vi "result text16be.vi"(7 "para3":u32, 8 "error in (no error)":errorcluster, 9 "para2":i32, 10 "para1":u32, 11 "para0":dbl) -> (0 "error out":errorcluster, 3 "para0 out":dbl, 5 "para3 out":u32)   [LabVIEW 2020, in "sqlite3.lvlib"]
uses:
  sqlite3.lvlib
  errstr.vi
  bin/sqlite3_64.dll
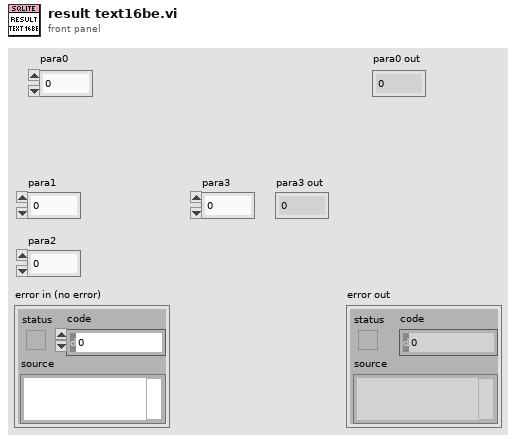
[diagram p1: front panel]
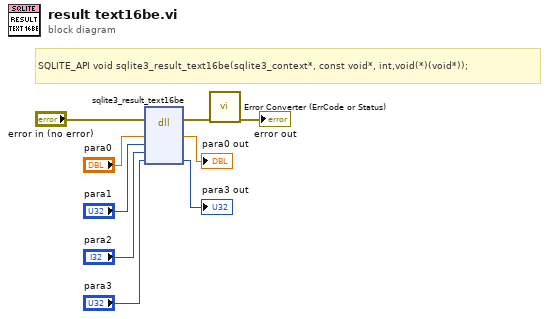
[diagram p0: block diagram]
diagram:
  # "SQLITE_API void sqlite3_result_text16be(sqlite3_context*, const void*, int,void(*)(void*));"
  n1 = dll-call lib="D:/Project/Labview-Projects/database-configuration/externals/sqlite3/Source/bin/sqlite3_*.*" fn="sqlite3_result_text16be"(error in="error in (no error)", "para0"="para0", "para1"="para1", "para2"="para2", "para3"="para3") -> (error out=w2:errorcluster, "para0"=→"para0 out":dbl, "para3"=→"para3 out":u32)  [unwired: 5 in, 1 out]
  n2 = call "Error Converter (ErrCode or Status).vi"("error in (no error)"=w2) -> ("error out"=→"error out":errorcluster)  [unwired: 10 in]
